vi "Generate Folder Structure.vi"(8 "error in (no error)":errorcluster, 10 "Report Directory in":path, 11 "Report Generator in":refnum<class "Report Generator.lvclass">) -> (0 "error out":errorcluster, 2 "Report Directory out":path, 3 "Report Generator out":refnum<class "Report Generator.lvclass">)   [LabVIEW 2020, in "Report Generator.lvclass"]
uses:
  Report Generator.lvclass
  Report Generator.lvclass/Report Generator.ctl
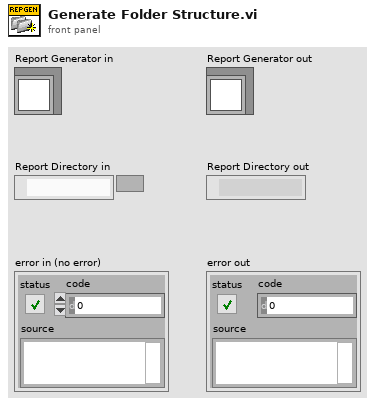
[diagram p1: front panel]
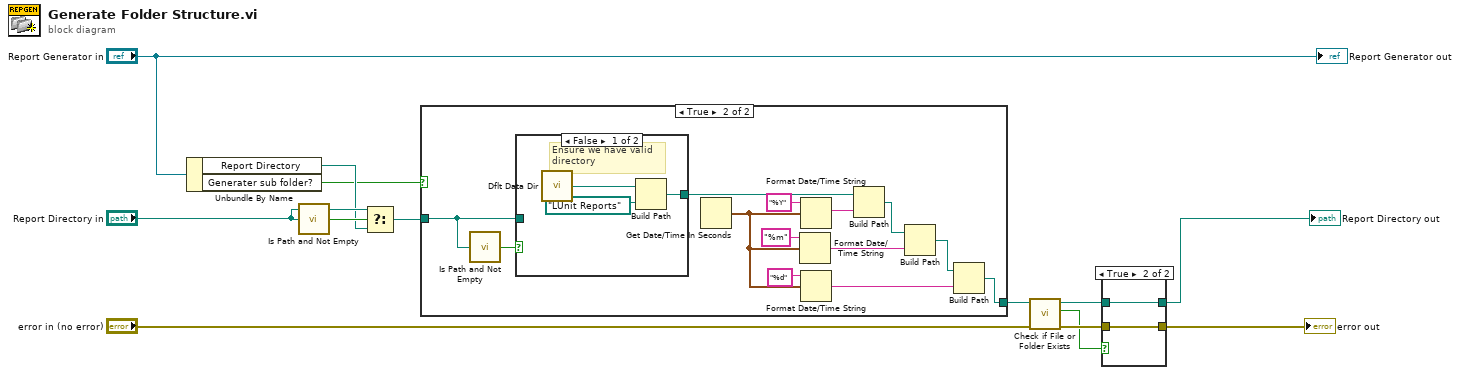
[diagram p0: block diagram]
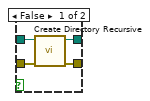
[diagram p4: hidden frame]
diagram:
  n1 = Unbundle By Name("Report Generator in") -> ("Report Directory"=w10:path, "Generater sub folder?"=w1:bool)
  n2 = call <vilib>:"Is Path and Not Empty.vi"("path"="Report Directory in") -> ("Is Path and Not Empty?"=w11:bool)  [unwired: 4 in]
  n3 = Select(t="Report Directory in", s=w11, f=w10) -> (s? t:f=w9:path)
  n4 = case shown="True" w1 {
    tunnel: w9 -> [w14 w27]
    tunnel: [w14 w17] -> w5
    frame False {
    }
    frame True {
      n5 = call <vilib>:"Is Path and Not Empty.vi"("path"=w27) -> ("Is Path and Not Empty?"=w16:bool)  [unwired: 4 in]
      n6 = case shown="False" w16 {
        tunnel: [w28 w31] -> w15
        tunnel: w27 -> [_ w31]
        frame False {
          # "Ensure we have valid \ndirectory"
          n7 = call <vilib>:"Dflt Data Dir.vi"() -> ("App:Default Data Directory"=w30:path)
          n8 = Build Path(base path=w30, name or relative path=path "LUnit Reports") -> (appended path=w28:path)
        }
        frame True {
        }
      }
      n9 = Get Date/Time In Seconds() -> (seconds since 1Jan1904=w22:timestamp)
      n10 = Format Date/Time String(time format string (%c)="%m", seconds (now)=w22) -> (date/time string=w19:string)  [unwired: 1 in]
      n11 = Format Date/Time String(time format string (%c)="%Y", seconds (now)=w22) -> (date/time string=w25:string)  [unwired: 1 in]
      n12 = Format Date/Time String(time format string (%c)="%d", seconds (now)=w22) -> (date/time string=w18:string)  [unwired: 1 in]
      n13 = Build Path(base path=w15, name or relative path=w25) -> (appended path=w21:path)
      n14 = Build Path(base path=w21, name or relative path=w19) -> (appended path=w20:path)
      n15 = Build Path(base path=w20, name or relative path=w18) -> (appended path=w17:path)
    }
  }
  n16 = call <vilib>:"Check if File or Folder Exists.vi"("error in (no error)"="error in (no error)", "path"=w5) -> ("error out"=w3:errorcluster, "file or folder exists?"=w2:bool, "dup path"=w4:path)  [unwired: 7 in]
  n17 = case shown="True" w2 {
    tunnel: [w35 w37] -> w8
    tunnel: [w34 w36] -> w7
    tunnel: w4 -> [w33 w37]
    tunnel: w3 -> [w32 w36]
    frame False {
      n18 = call <vilib>:"Create Directory Recursive.vi"("error in (no error)"=w32, "directory"=w33) -> ("error out"=w34:errorcluster, "directory copy"=w35:path)  [unwired: 3 in, 1 out]
    }
    frame True {
    }
  }
  "error out" <- w7
  "Report Directory out" <- w8
  "Report Generator out" <- "Report Generator in"
